vi "GetHelium.vi"(6 "error in (no error)":errorcluster, 7 "Instrument Refnum in":refnum<k24>) -> (1 "Helium Level (%)":dbl, 2 "error out":errorcluster, 3 "Instrument Ref Out":refnum<k24>)   [LabVIEW 2016]
uses:
  C:/user/patrick/hg/levylab_inst_ppms2/lvsrc/PPMS2/QDInstrument_LabView/QDInstrument.dll
  QDInstrument.dll
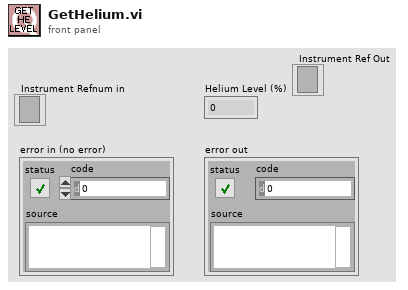
[diagram p1: front panel]
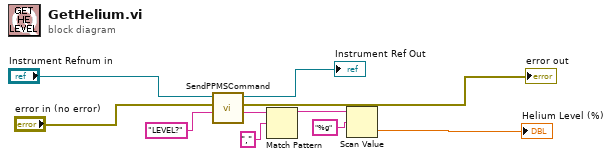
[diagram p0: block diagram]
diagram:
  n1 = call "SendPPMSCommand.vi"("PpmsCommand"="LEVEL?", "error in (no error)"="error in (no error)", "Instrument Ref In"="Instrument Refnum in") -> ("PpmsReply"=w9:string, "error out"=→"error out":errorcluster, "Instrument Ref Out"=→"Instrument Ref Out":refnum<k24>)  [unwired: 4 in, 2 out]
  n2 = Match Pattern(string=w9, regular expression=",") -> (before substring=w7:string)  [unwired: 1 in, 3 out]
  n3 = Scan Value(string=w7, format string="%g") -> (value=→"Helium Level (%)":dbl)  [unwired: 1 in, 1 out]
